vi "Ej 9 Filtro_EMA.vi"() -> ()   [LabVIEW 2021]
panel:
  out "Array":dbl[](array[numeric])
  in  "x":dbl
  out "appended array":dbl[](array[numeric])
  in  "stop":bool
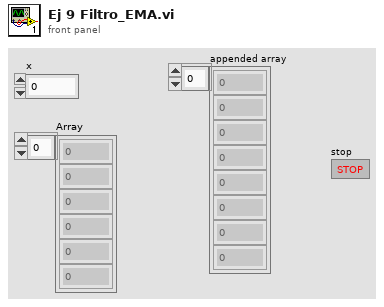
[diagram p1: front panel]
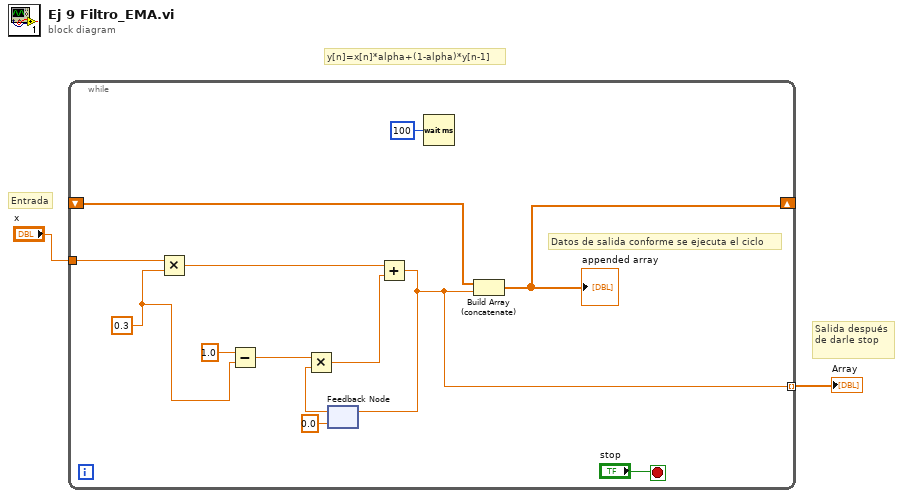
[diagram p0: block diagram]
diagram:
  # "y[n]=x[n]*alpha+(1-alpha)*y[n-1]"
  # "Salida después de darle stop"
  # "Entrada"
  n1 = while {
    shift-right: [w6] -> _
    shift-left: _ -> [w5]
    tunnel: [w4] -> w2 mode=indexing
    tunnel: "x" -> [w3]
    stop <- "stop" stop-if-true
    w11 = 0.3 ("y")
    # "Datos de salida conforme se ejecuta el ciclo"
    n2 = Multiply(x=w3, y=w11) -> (x*y=w13:dbl)
    n3 = Subtract(x=1.0, y=w11) -> (x-y=w10:dbl)
    n4 = feedback #1(0.0) -> (w8:dbl)
    n5 = Multiply(x=w10, y=w8) -> (x*y=w9:dbl)
    n6 = Add(x=w13, y=w9) -> (x+y=w4:dbl)
    n7 = feedback-in #1(w4) -> ()
    n8 = Wait (ms)(milliseconds to wait=u32 100) -> ()  [unwired: 1 out]
    n9 = Build Array (concatenate)(w5, w4) -> (w6:dbl[])
    "appended array" <- w6
  }
  "Array" <- w2
